vi "NoColisionManMarkerWithCenterBack.vi"(10 "Pos ManMarker":dbl[](array[numeric]) format="%#_13g", 11 "Pos CenterBacks":dbl[][](array[numeric]) format="%#_13g") -> (3 "Pos ManMarker":dbl[](array[numeric]) format="%#_13g")   [LabVIEW 2017]
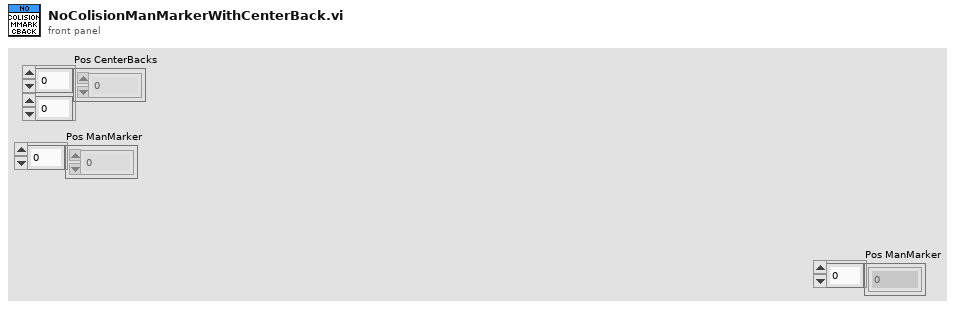
[diagram p1: front panel]
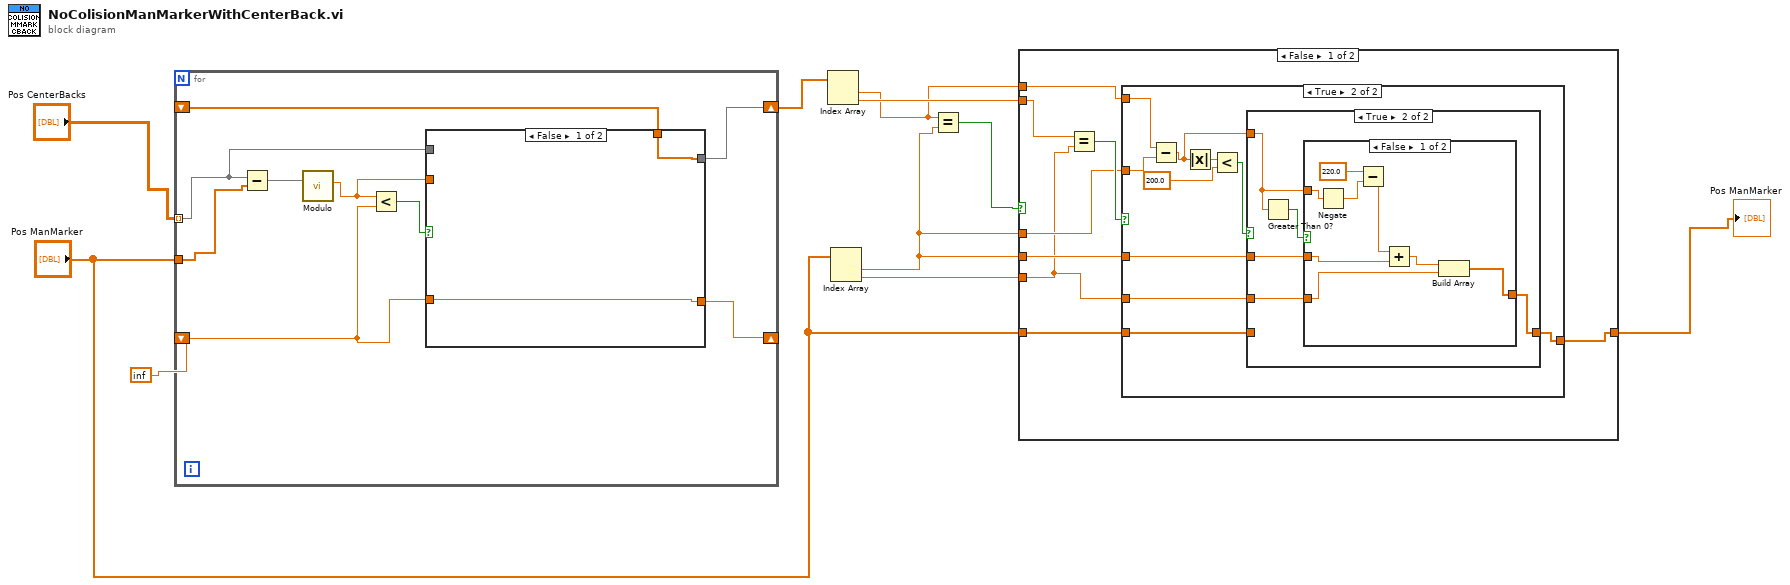
[diagram p0: block diagram]
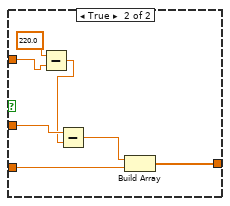
[diagram p4: hidden frame]
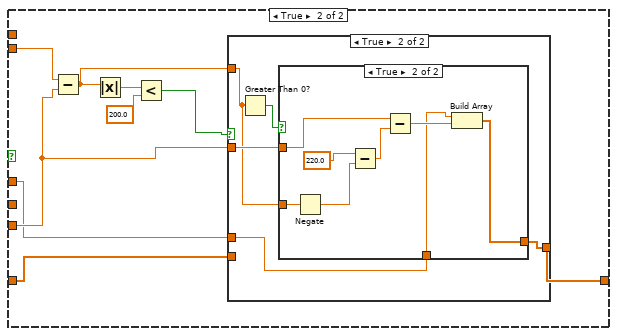
[diagram p5: hidden frame]
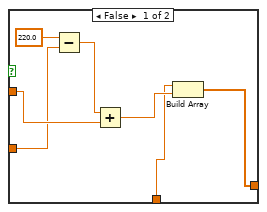
[diagram p7: hidden frame]
diagram:
  n1 = for {
    tunnel: "Pos CenterBacks" -> [w13] mode=indexing
    tunnel: "Pos ManMarker" -> [w19]
    shift-right: [w16] -> _
    shift-left: inf -> [w11]
    shift-right: [w14] -> w8
    shift-left: _ -> [w12]
    n2 = Subtract(x=w13, y=w19) -> (x-y=w18:dbl[])
    n3 = call "Modulo.vi"("2D vector"=w18) -> ("Modulo"=w15:dbl)  [unwired: 10 in]
    n4 = Less?(x=w15, y=w11) -> (x < y?=w17:bool)
    n5 = case shown="False" w17 {
      tunnel: [w21 w23] -> w16
      tunnel: w15 -> [_ w23]
      tunnel: w11 -> [w21 _]
      tunnel: [w20 w22] -> w14
      tunnel: w13 -> [_ w22]
      tunnel: w12 -> [w20 _]
      frame False {
      }
      frame True {
      }
    }
  }
  n6 = Index Array(array=w8) -> (element #1=w2:dbl, element #2=w6:dbl)  [unwired: 2 in]
  n7 = Index Array(array="Pos ManMarker") -> (element #1=w1:dbl, element #2=w5:dbl)  [unwired: 2 in]
  n8 = Equal?(x=w2, y=w1) -> (x = y?=w7:bool)
  n9 = case shown="False" w7 {
    tunnel: w6 -> [w31 w72]
    tunnel: w5 -> [w24 w66]
    tunnel: [w29 w68] -> w4
    tunnel: "Pos ManMarker" -> [w28 w67]
    tunnel: w1 -> [w26 w64]
    tunnel: w2 -> [w27 _]
    tunnel: w1 -> [w25 _]
    frame False {
      n10 = Equal?(x=w31, y=w24) -> (x = y?=w30:bool)
      n11 = case shown="True" w30 {
        tunnel: [w32 w38] -> w29
        tunnel: w28 -> [w32 w37]
        tunnel: w27 -> [_ w42]
        tunnel: w26 -> [_ w41]
        tunnel: w25 -> [_ w34]
        tunnel: w24 -> [_ w33]
        frame False {
        }
        frame True {
          n12 = Subtract(x=w42, y=w41) -> (x-y=w35:dbl)
          n13 = Absolute Value(x=w35) -> (abs(x)=w36:dbl)
          n14 = Less?(x=w36, y=200.0) -> (x < y?=w39:bool)
          n15 = case shown="True" w39 {
            tunnel: [w43 w45] -> w38
            tunnel: w37 -> [w43 _]
            tunnel: w35 -> [_ w46]
            tunnel: w34 -> [_ w47]
            tunnel: w33 -> [_ w44]
            frame False {
            }
            frame True {
              n16 = Greater Than 0?(x=w46) -> (x > 0?=w48:bool)
              n17 = case shown="False" w48 {
                tunnel: w47 -> [w56 w63]
                tunnel: w46 -> [w54 w61]
                tunnel: [w51 w58] -> w45
                tunnel: w44 -> [w49 w57]
                frame False {
                  n18 = Negate(x=w54) -> (-x=w53:dbl)
                  n19 = Subtract(x=220.0, y=w53) -> (x-y=w52:dbl)
                  n20 = Add(x=w52, y=w56) -> (x+y=w50:dbl)
                  n21 = Build Array(w50, w49) -> (w51:dbl[])
                }
                frame True {
                  n22 = Subtract(x=220.0, y=w61) -> (x-y=w60:dbl)
                  n23 = Subtract(x=w63, y=w60) -> (x-y=w59:dbl)
                  n24 = Build Array(w59, w57) -> (w58:dbl[])
                }
              }
            }
          }
        }
      }
    }
    frame True {
      n25 = Subtract(x=w72, y=w66) -> (x-y=w65:dbl)
      n26 = Absolute Value(x=w65) -> (abs(x)=w71:dbl)
      n27 = Less?(x=w71, y=200.0) -> (x < y?=w69:bool)
      n28 = case shown="True" w69 {
        tunnel: [w73 w75] -> w68
        tunnel: w67 -> [w73 _]
        tunnel: w65 -> [_ w74]
        tunnel: w66 -> [_ w77]
        tunnel: w64 -> [_ w76]
        frame False {
        }
        frame True {
          n29 = Greater Than 0?(x=w74) -> (x > 0?=w78:bool)
          n30 = case shown="True" w78 {
            tunnel: w77 -> [w85 w93]
            tunnel: w74 -> [w83 w87]
            tunnel: w76 -> [w80 w89]
            tunnel: [w79 w88] -> w75
            frame False {
              n31 = Subtract(x=220.0, y=w83) -> (x-y=w82:dbl)
              n32 = Add(x=w82, y=w85) -> (x+y=w81:dbl)
              n33 = Build Array(w80, w81) -> (w79:dbl[])
            }
            frame True {
              n34 = Negate(x=w87) -> (-x=w86:dbl)
              n35 = Subtract(x=220.0, y=w86) -> (x-y=w91:dbl)
              n36 = Subtract(x=w93, y=w91) -> (x-y=w90:dbl)
              n37 = Build Array(w89, w90) -> (w88:dbl[])
            }
          }
        }
      }
    }
  }
  "Pos ManMarker" <- w4
